vi "Shooter.vi"(11 "Shooter":bool) -> ()   [LabVIEW 2017]
uses:
  Robot Global Data.vi
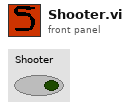
[diagram p1: front panel]
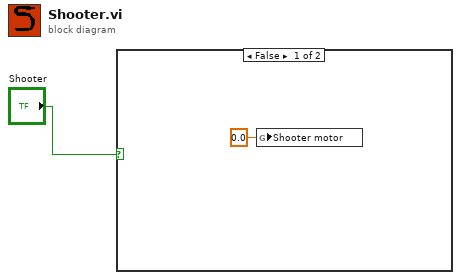
[diagram p0: block diagram]
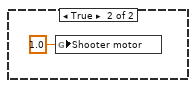
[diagram p2: hidden frame]
diagram:
  n1 = case shown="False" "Shooter" {
    frame False {
      n2 = global write "Robot Global Data.vi" "Shooter motor"(0.0 ("Shooter motor")) -> ()
    }
    frame True {
      n3 = global write "Robot Global Data.vi" "Shooter motor"(1.0 ("Shooter motor")) -> ()
    }
  }
